vi "Keithley2182AMonitor.vi"() -> ()   [LabVIEW 2019]
uses:
  Utility/Monitor Communication/K2812A/K2812A_cluster.ctl
  Equipment/Keithley 622x/Configure/2182 -A/Low Level/Typedefs/KE2182 -- Voltage Ranges.ctl
  Global/Global Variables/Data_Display_global.vi
  Instrument_Setup.vi
  <vilib>/ErrorRing/Error Ring.xnode
  Equipment/Keithley 2182/Keithley 2182.lvlib
  Equipment/Keithley 622x/Keithley 622x.lvlib
panel:
  in  "stop":bool
  out "K2182A Cluster":T1
  # "K 2182A"
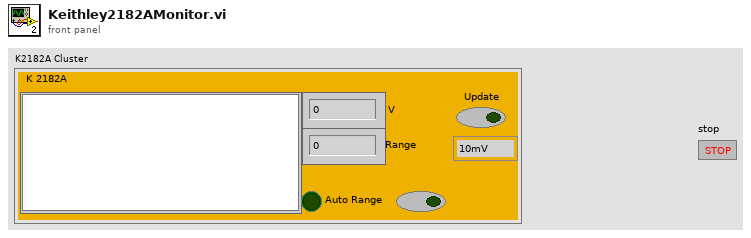
[diagram p1: front panel]
types:
  T1 = typedef "K2812A_cluster.ctl" = cluster{"Plot Window":dbl[][], "Range":dbl, "Update":bool, "Range selector":T2, "Auto Range":bool, "V":dbl, "Auto Range set":bool}
  T2 = typedef "Keithley 622x.lvlib/KE2182 -- Voltage Ranges.ctl" = enum16{"10mV", "100mV", "1V", "10V", "100V"}
  T3 = cluster{"VISA Keithley 2182A":refnum<visa-resource-name>, "Measurement (0: Voltage Channel 1)":i32, "Integration Rate (5)":dbl, "Integration Rate Units (0: Line Cycles)":i32, "Sample Count (1)":i32, "Voltage Resolution (8)":i32, "Enable Ratio (F: Disable)":bool, "Enable Delta (F: Disable)":bool, "Enable Analog Filter (T: Enable)":bool, "Enable Digital Filter (T: Enable)":bool, "Filter Window (0.01%)":dbl, "Filter Count (10)":i32, "Filter Type (0: Moving)":i32}
  T4 = typedef "K2812A_control.ctl" = cluster{"Update":bool, "Range selector":T2, "Auto Range":bool}
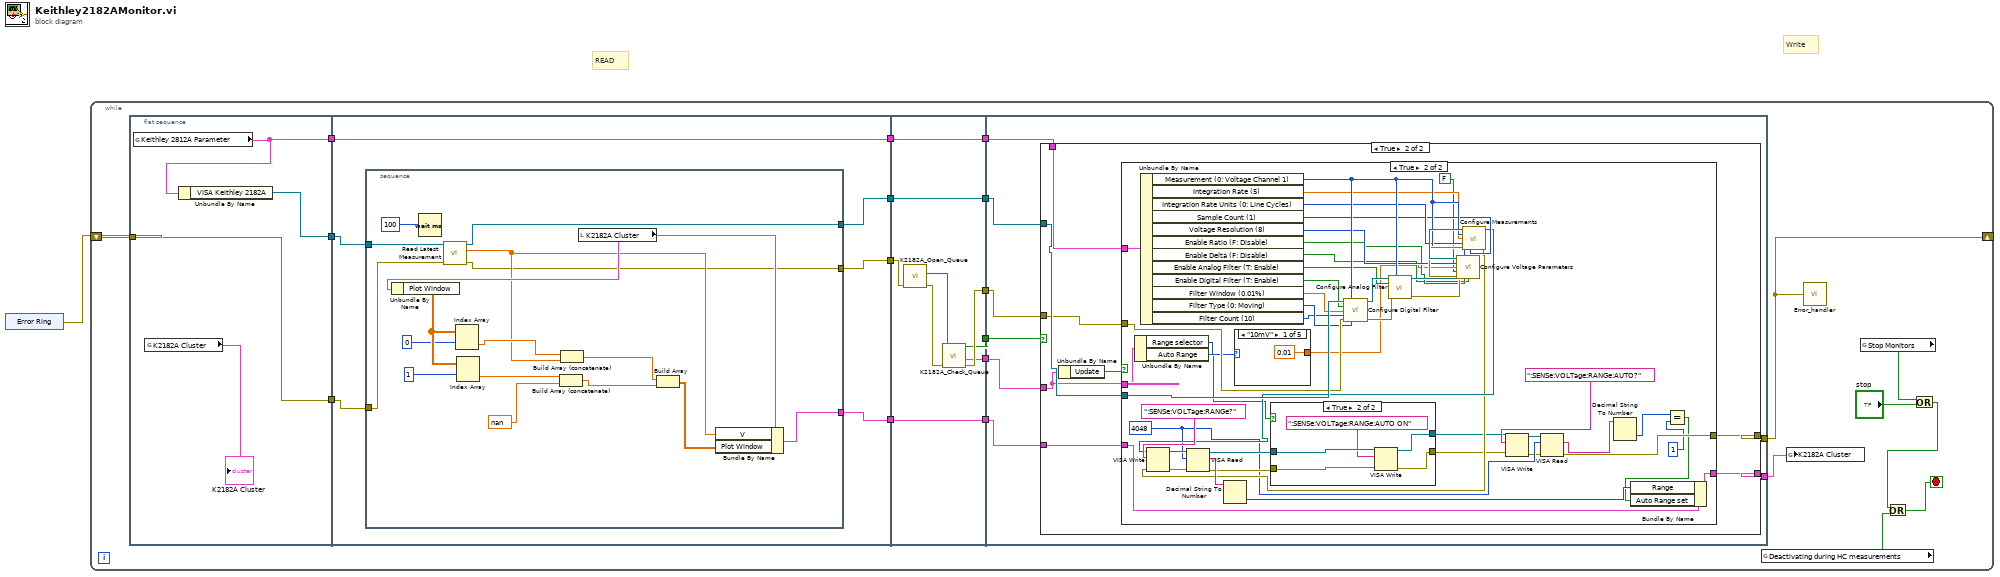
[diagram p0: block diagram]
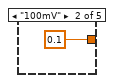
[diagram p5: hidden frame]
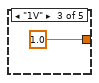
[diagram p6: hidden frame]
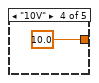
[diagram p7: hidden frame]
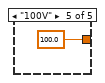
[diagram p8: hidden frame]
diagram:
  # "Write"
  # "READ"
  n1 = xnode "Error Ring"() -> ("error out"=w1:errorcluster)
  n2 = while {
    shift-right: [w6] -> _
    shift-left: w1 -> [w20]
    stop <- w21 stop-if-true
    n3 = flat-sequence {
      tunnel: w20 -> [w24]
      tunnel: [w26] -> w19
      tunnel: [w25] -> w18
      tunnel: [w24] -> w17
      tunnel: w19 -> [w32]
      tunnel: w18 -> [w31]
      tunnel: w17 -> [w30]
      tunnel: [w32] -> w16
      tunnel: [w29] -> w15
      tunnel: [w28] -> w14
      tunnel: [w27] -> w13
      tunnel: w16 -> [w58]
      tunnel: w15 -> [w57]
      tunnel: w14 -> [w53]
      tunnel: w13 -> [w56]
      tunnel: [w58] -> w12
      tunnel: [w57] -> w11
      tunnel: [w56] -> w10
      tunnel: [w52] -> w9
      tunnel: [w51] -> w8
      tunnel: [w50] -> w7
      tunnel: w12 -> [w62]
      tunnel: w11 -> [w61]
      tunnel: w10 -> [w63]
      tunnel: w9 -> [w65]
      tunnel: w8 -> [w64]
      tunnel: w7 -> [w66]
      tunnel: [w60] -> w6
      tunnel: [w59] -> w5
      frame #0 {
        n4 = global read "Instrument_Setup.vi" "Keithley 2812A Parameter"() -> (w26:T3)
        n5 = global read "Data_Display_global.vi" "K2182A Cluster"() -> (→"K2182A Cluster":T1)
        n6 = Unbundle By Name(w26) -> ("VISA Keithley 2182A"=w25:refnum<visa-resource-name>)
      }
      frame #1 {
        n7 = stacked-sequence {
          tunnel: w31 -> [w48]
          tunnel: w30 -> [w47]
          tunnel: [w35] -> w29
          tunnel: [w34] -> w28
          tunnel: [w33] -> w27
          frame #0 {
            n8 = Wait (ms)(milliseconds to wait=100) -> ()  [unwired: 1 out]
            n9 = call "Read Latest Measurement.vi"("error in (no error)"=w47, "VISA resource name"=w48) -> ("error out"=w34:errorcluster, "Measurement"=w41:dbl, "VISA resource name out"=w33:refnum<visa-resource-name>)  [unwired: 6 in, 1 out]
            n10 = local read "K2182A Cluster"() -> (w46:T1)
            n11 = Unbundle By Name(w46) -> ("Plot Window"=w45:dbl[][])
            n12 = Index Array(array=w45, index (row)=0) -> (element=w42:dbl[])  [unwired: 1 in]
            n13 = Index Array(array=w45, index (row)=1) -> (element=w40:dbl[])  [unwired: 1 in]
            n14 = Build Array (concatenate)(w40, nan) -> (w38:dbl[])
            n15 = Build Array (concatenate)(w42, w41) -> (w37:dbl[])
            n16 = Build Array(w37, w38) -> (w36:dbl[][])
            n17 = Bundle By Name(cluster=w46, "V"=w41, "Plot Window"=w36) -> (w35:T1)
          }
        }
      }
      frame #2 {
        n18 = call "K2182A_Open_Queue.vi"("error in (no error)"=w53) -> ("error out"=w54:errorcluster, "queue out"=w55:refnum<queue>)  [unwired: 9 in]
        n19 = call "K2182A_Check_Queue.vi"("error in (no error)"=w54, "queue"=w55) -> ("error out"=w52:errorcluster, "Control"=w51:T4, "New Entries?"=w50:bool)  [unwired: 6 in]
      }
      frame #3 {
        n20 = case shown="True" w66 {
          tunnel: w65 -> [w68 w75]
          tunnel: w64 -> [_ w74]
          tunnel: w63 -> [_ w76]
          tunnel: [w68 w73] -> w60
          tunnel: w62 -> [_ w72]
          tunnel: w61 -> [w67 w71]
          tunnel: [w67 w70] -> w59
          frame False {
          }
          frame True {
            n21 = Unbundle By Name(w74) -> ("Update"=w69:bool)
            n22 = case shown="True" w69 {
              tunnel: w76 -> [_ w124]
              tunnel: w75 -> [w78 w120]
              tunnel: w74 -> [_ w125]
              tunnel: [w78 w83] -> w73
              tunnel: w72 -> [_ w126]
              tunnel: w71 -> [w77 w102]
              tunnel: [w77 w101] -> w70
              frame False {
              }
              frame True {
                w89 = u32 4048 ("byte count")
                n23 = Unbundle By Name(w125) -> ("Range selector"=w108:T2, "Auto Range"=w92:bool)
                n24 = Unbundle By Name(w126) -> ("Measurement (0: Voltage Channel 1)"=w116:i32, "Integration Rate (5)"=w115:dbl, "Integration Rate Units (0: Line Cycles)"=w114:i32, "Sample Count (1)"=w113:i32, "Voltage Resolution (8)"=w112:i32, "Enable Ratio (F: Disable)"=w111:bool, "Enable Delta (F: Disable)"=w110:bool, "Enable Analog Filter (T: Enable)"=w109:bool, "Enable Digital Filter (T: Enable)"=w106:bool, "Filter Window (0.01%)"=w105:dbl, "Filter Type (0: Moving)"=w104:i32, "Filter Count (10)"=w103:i32)
                n25 = case shown="\"10mV\"" w108 {
                  tunnel: [0.01 0.1 1.0 10.0 100.0] -> w107
                  frame "10mV" {
                  }
                  frame "100mV" {
                  }
                  frame "1V" {
                  }
                  frame "10V" {
                  }
                  frame "100V" {
                  }
                }
                n26 = call "Configure Digital Filter.vi"("VISA resource name"=w124, "Measurement (0: Voltage Channel 1)"=w116, "Enable Digital Filter (T: Enable)"=w106, "Filter Window (0.01%)"=w105, "Filter Count (10)"=w103, "error in (no error)"=w120, "Filter Type (0: Moving)"=w104) -> ("VISA resource name out"=w123:refnum<visa-resource-name>, "error out"=w119:errorcluster)  [unwired: 7 in]
                n27 = call "Configure Analog Filter.vi"("VISA resource name"=w123, "Measurement (0: Voltage Channel 1)"=w116, "Enable Analog Filter (T: Enable)"=w109, "error in (no error)"=w119) -> ("VISA resource name out"=w122:refnum<visa-resource-name>, "error out"=w118:errorcluster)  [unwired: 10 in]
                n28 = call "Configure Voltage Parameters.vi"("VISA resource name"=w122, "Measurement (1: Voltage Channel 1)"=w116, "Voltage Resolution (8)"=w112, "Range Value (12)"=w107, "Autorange (T: Enable)"=FALSE, "error in (no error)"=w118, "Enable Ratio (F: Disable)"=w111, "Enable Delta (F: Disable)"=w110) -> ("VISA resource name out"=w121:refnum<visa-resource-name>, "error out"=w117:errorcluster)  [unwired: 6 in]
                n29 = call "Configure Measurements.vi"("VISA resource name"=w121, "Measurement (0: Voltage Channel 1)"=w116, "Integration Rate (5)"=w115, "Integration Rate Units (0: Line Cycles)"=w114, "error in (no error)"=w117, "Sample Count (1)"=w113) -> ("VISA resource name out"=w94:refnum<visa-resource-name>, "error out"=w93:errorcluster)  [unwired: 8 in]
                n30 = VISA Write(VISA resource name=w94, write buffer=":SENSe:VOLTage:RANGe?", error in (no error)=w93) -> (VISA resource name out=w99:refnum<visa-resource-name>, error out=w98:errorcluster)  [unwired: 1 out]
                n31 = VISA Read(VISA resource name=w99, byte count=w89, error in (no error)=w98) -> (VISA resource name out=w91:refnum<visa-resource-name>, read buffer=w97:string, error out=w90:errorcluster)  [unwired: 1 out]
                n32 = Decimal String To Number(string=w97) -> (number=w96:i32)  [unwired: 2 in, 1 out]
                n33 = case shown="True" w92 {
                  tunnel: w91 -> [w128 w133]
                  tunnel: w90 -> [w127 w132]
                  tunnel: [w128 w130] -> w87
                  tunnel: [w127 w129] -> w85
                  frame False {
                  }
                  frame True {
                    n34 = VISA Write(VISA resource name=w133, write buffer=":SENSe:VOLTage:RANGe:AUTO ON", error in (no error)=w132) -> (VISA resource name out=w130:refnum<visa-resource-name>, error out=w129:errorcluster)  [unwired: 1 out]
                  }
                }
                n35 = VISA Write(VISA resource name=w87, write buffer=":SENSe:VOLTage:RANGe:AUTO?", error in (no error)=w85) -> (VISA resource name out=w86:refnum<visa-resource-name>, error out=w84:errorcluster)  [unwired: 1 out]
                n36 = VISA Read(VISA resource name=w86, byte count=w89, error in (no error)=w84) -> (read buffer=w82:string, error out=w83:errorcluster)  [unwired: 2 out]
                n37 = Decimal String To Number(string=w82) -> (number=w81:i32)  [unwired: 2 in, 1 out]
                n38 = Equal?(x=w81, y=1) -> (x = y?=w79:bool)
                n39 = Bundle By Name(cluster=w102, "Range"=w96, "Auto Range set"=w79) -> (w101:T1)
              }
            }
          }
        }
      }
    }
    n40 = global read "Data_Display_global.vi" "Deactivating during HC measurements"() -> (w22:bool)
    n41 = global write "Data_Display_global.vi" "K2182A Cluster"(w5) -> ()
    n42 = call "Error_handler.vi"("error constant"=w6) -> ()
    n43 = global read "Data_Display_global.vi" "Stop Monitors"() -> (w4:bool)
    n44 = Or(x=w4, y="stop") -> (x .or. y?=w2:bool)
    n45 = Or(x=w2, y=w22) -> (x .or. y?=w21:bool)
  }
